vi "acceptCommand.vi"() -> ()   [LabVIEW 2016, in "Commands.lvlib" / "Enable.lvclass"]
uses:
  Enable.lvclass
  MiddlewareSALThisComponent/MiddlewareSALThisComponent.lvclass
panel:
  out "MiddlewareSALThisComponent out":refnum<class "MiddlewareSALThisComponent.lvclass">
  in  "MiddlewareSALThisComponent in":refnum<class "MiddlewareSALThisComponent.lvclass">
  out "error out":errorcluster
  in  "error in (no error)":errorcluster
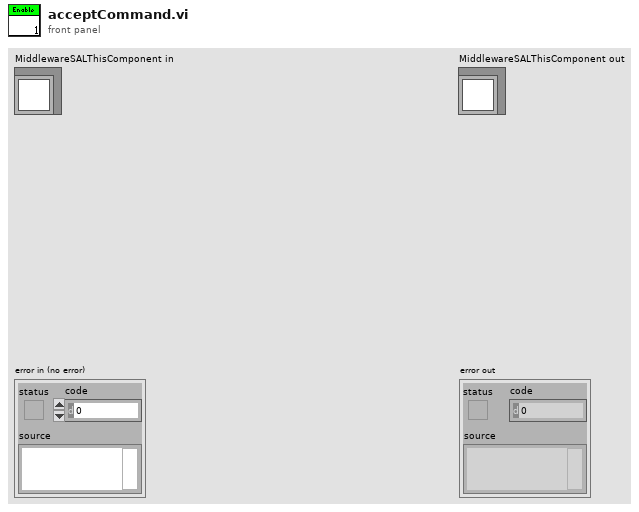
[diagram p1: front panel]
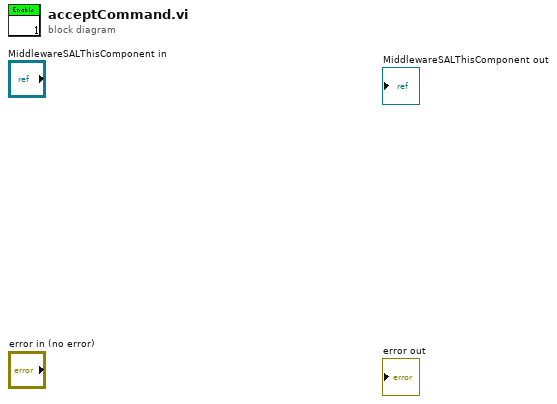
[diagram p0: block diagram]
diagram:
